vi "SOUR_POW_CORR_COLL_TABL_DATA.vi"(0 "VISA IN":refnum<visa-resource-name>, 5 "error in":errorcluster, 7 "Channel":i32) -> (14 "VISA Out":refnum<visa-resource-name>, 19 "error out":errorcluster)   [LabVIEW 2018, in "PNA-X.lvlib"]
doc: "SOURce:POWer:CORRection:COLLect:TABLe:DATA"
uses:
  PNA-X.lvlib
panel:
  in  "Data":string
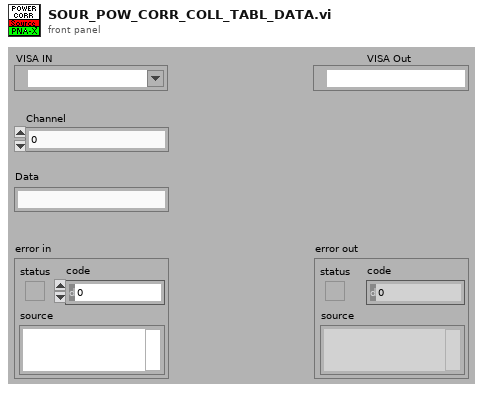
[diagram p1: front panel]
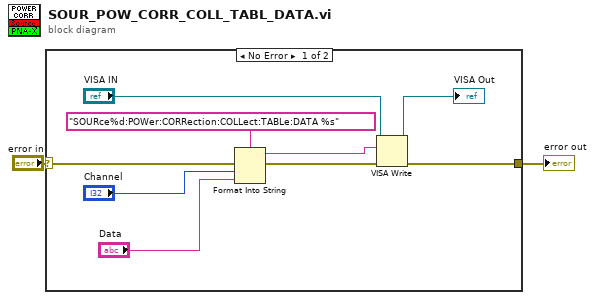
[diagram p0: block diagram]
diagram:
  n1 = case shown="No Error" "error in" {
    selector: "error in" -> [w8 w12]
    tunnel: [w10 w12] -> w1
    frame No Error {
      n2 = Format Into String(format string="SOURce%d:POWer:CORRection:COLLect:TABLe:DATA %s" ("Cmdline"), error in=w8, "Channel", "Data") -> (resulting string=w3:string, error out=w7:errorcluster)  [unwired: 1 in]
      n3 = VISA Write(VISA resource name="VISA IN", write buffer=w3, error in (no error)=w7) -> (VISA resource name out=→"VISA Out":refnum<visa-resource-name>, error out=w10:errorcluster)  [unwired: 1 out]
    }
    frame Error {
    }
  }
  "error out" <- w1
